vi "Spex StartScan.vi"(6 "Moving Ref":refnum<vi>, 8 "error in":errorcluster, 9 "Lambda Ref":refnum<vi>, 10 "Scan Type":bool, 11 "Port":refnum<visa-resource-name>="COM1" caption="Com Port") -> (0 "error out":errorcluster, 2 "SpexOut":string caption="Spex Output", 3 "Wlenght":dbl caption="Wavelenght (nm)")   [LabVIEW 2019]
doc: "Ce Vi envoie la commande de Scan au monochromateur SPEX.\n\nScan Type: définit le mode de balayage. True: Normal, False:Trigger"
uses:
  <userlib>/GenProg/WritebyWeakRefBool.vi
  <vilib>/Instr/_visa.llb/VISA Configure Serial Port (Instr).vi
  <userlib>/GenProg/WritebyWeakRefNum.vi
panel:
  out "Port Out":refnum<visa-resource-name>="COM1" caption="Com Port"
  # "Normal"
  # "Trigger"
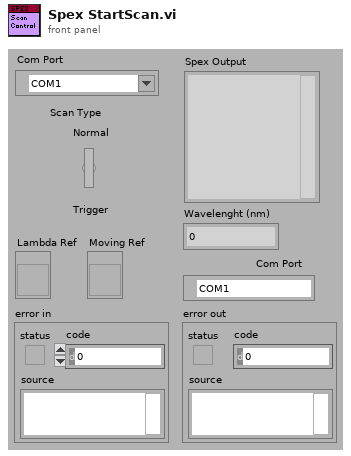
[diagram p1: front panel]
types:
  T1 = enum16{"Start Scan", "Wait Answer", "Wait Start", "Error"}
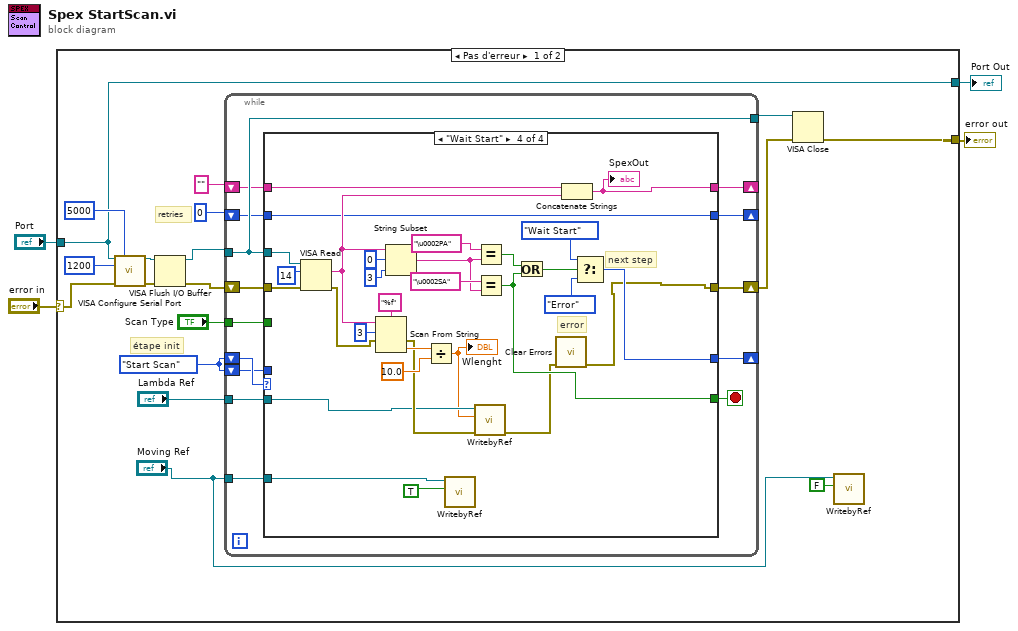
[diagram p0: block diagram]
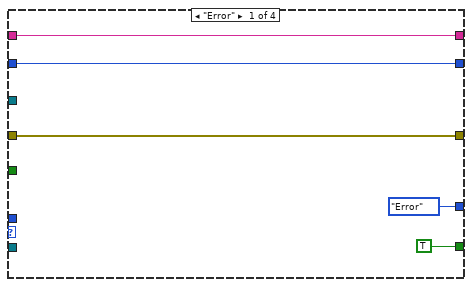
[diagram p2: hidden frame]
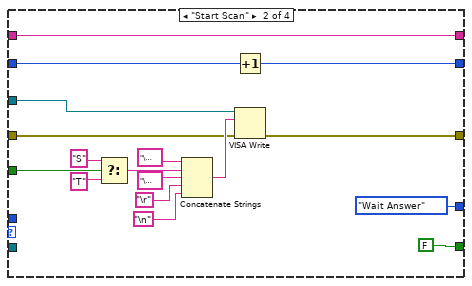
[diagram p3: hidden frame]
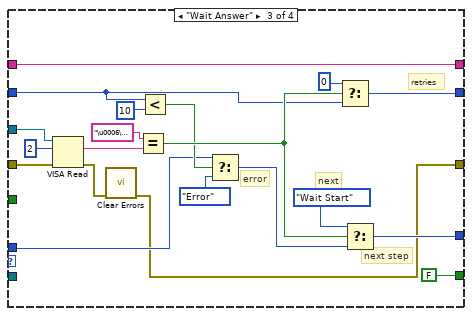
[diagram p4: hidden frame]
diagram:
  n1 = case shown="Pas d'erreur" "error in" {
    selector: "error in" -> [w10 w110]
    tunnel: [w9 w110] -> w3
    tunnel: [w8 w109] -> w2
    tunnel: "Port" -> [w8 w109]
    frame No Error {
      w14 = T1."Start Scan"
      # "retries"
      # "étape init"
      n2 = call-poly "VISA Configure Serial Port"("VISA resource name"=w8, "timeout (10sec)"=u32 5000, "baud rate (9600)"=u32 1200, "error in (no error)"=w10) -> ("VISA resource name out"=w19:refnum<visa-resource-name>, "error out"=w20:errorcluster)  [unwired: 10 in]
      n3 = VISA Flush I/O Buffer(VISA resource name=w19, error in (no error)=w20) -> (VISA resource name out=w17:refnum<visa-resource-name>, error out=w18:errorcluster)  [unwired: 1 in]
      n4 = while {
        shift-right: [w28] -> _
        shift-left: w14 -> [w36]
        tunnel: w17 -> [w32]
        shift-right: [w34] -> w11
        shift-left: w18 -> [w35]
        tunnel: [w32] -> w12
        shift-right: [w30] -> _
        shift-left: 0 -> [w31]
        shift-left: w14 -> [w29]
        tunnel: "Scan Type" -> [w27]
        shift-right: [w25] -> _
        shift-left: "" -> [w26]
        tunnel: "Lambda Ref" -> [w24]
        tunnel: "Moving Ref" -> [w23]
        stop <- w33 stop-if-true
        n5 = case shown="\"Wait Start\"" w36 {
          tunnel: w32 -> [_ w53 w76 w107]
          tunnel: w35 -> [w37 w52 w75 w87]
          tunnel: [w37 w51 w59 w86] -> w34
          tunnel: [T1."Error" T1."Wait Answer" w77 w92] -> w28
          tunnel: [TRUE FALSE FALSE w85] -> w33
          tunnel: w31 -> [w40 w49 w70 w91]
          tunnel: [w40 w48 w66 w91] -> w30
          tunnel: w29 -> [_ _ w64 _]
          tunnel: w27 -> [_ w45 _ _]
          tunnel: w26 -> [w38 w42 w61 w100]
          tunnel: [w38 w42 w61 w98] -> w25
          tunnel: w24 -> [_ _ _ w82]
          tunnel: w23 -> [_ _ _ w81]
          frame "Error" {
          }
          frame "Start Scan" {
            n6 = Select(t="S" ("initial string"), s=w45, f="T" ("initial string")) -> (s? t:f=w44:string)
            n7 = Concatenate Strings("\u0018" ("string"), w44, "\u0003" ("string"), "\r", "\n") -> (w54:string)
            n8 = Increment(x=w49) -> (x+1=w48:i32)
            n9 = VISA Write(VISA resource name=w53, write buffer=w54, error in (no error)=w52) -> (error out=w51:errorcluster)  [unwired: 2 out]
          }
          frame "Wait Answer" {
            # "next"
            # "error"
            # "next step"
            # "retries"
            n10 = VISA Read(VISA resource name=w76, byte count=u32 2, error in (no error)=w75) -> (read buffer=w73:string, error out=w60:errorcluster)  [unwired: 2 out]
            n11 = call <vilib>:"Clear Errors.vi"("error in (no error)"=w60) -> ("error out"=w59:errorcluster)  [unwired: 5 in, 1 out]
            n12 = Equal?(x="\u0006\u0018", y=w73) -> (x = y?=w71:bool)
            n13 = Less?(x=w70, y=10) -> (x < y?=w68:bool)
            n14 = Select(t=w64, s=w68, f=T1."Error") -> (s? t:f=w67:T1)
            n15 = Select(t=0, s=w71, f=w70) -> (s? t:f=w66:i32)
            n16 = Select(t=T1."Wait Start", s=w71, f=w67) -> (s? t:f=w77:T1)
          }
          frame "Wait Start" {
            # "error"
            # "next step"
            n17 = VISA Read(VISA resource name=w107, byte count=u32 14, error in (no error)=w87) -> (read buffer=w99:string, error out=w89:errorcluster)  [unwired: 2 out]
            n18 = Scan From String(format string="%f", input string=w99, initial scan location=u32 3, error in=w89) -> (error out=w84:errorcluster, output 1=w101:dbl)  [unwired: 1 in, 2 out]
            n19 = String Subset(string=w99, offset (0)=0, length (rest)=3 ("length (rest)")) -> (substring=w96:string)
            n20 = Divide(x=w101, y=10.0) -> (x/y=w79:dbl)
            "Wlenght" <- w79
            n21 = call-poly <userlib>:"WritebyRef.vi"("Valeur"=TRUE, "Control Ref"=w81) -> ()  [unwired: 9 in, 1 out]
            n22 = call-poly <userlib>:"WritebyRef.vi"("error in"=w84, "Valeur"=w79, "Control Ref"=w82) -> ("error out"=w83:errorcluster)  [unwired: 8 in]
            n23 = Equal?(x="\u0002PA", y=w96) -> (x = y?=w95:bool)
            n24 = Equal?(x="\u0002SA", y=w96) -> (x = y?=w85:bool)
            n25 = Or(x=w95, y=w85) -> (x .or. y?=w94:bool)
            n26 = call <vilib>:"Clear Errors.vi"("error in (no error)"=w83) -> ("error out"=w86:errorcluster)  [unwired: 5 in, 1 out]
            n27 = Concatenate Strings(w100, w99) -> (w98:string)
            "SpexOut" <- w98
            n28 = Select(t=T1."Wait Start", s=w94, f=T1."Error") -> (s? t:f=w92:T1)
          }
        }
      }
      n29 = VISA Close(VISA resource name=w12, error in (no error)=w11) -> (error out=w9:errorcluster)
      n30 = call-poly <userlib>:"WritebyRef.vi"("Valeur"=FALSE, "Control Ref"="Moving Ref") -> ()  [unwired: 9 in, 1 out]
    }
    frame Error {
    }
  }
  "error out" <- w3
  "Port Out" <- w2
